vi "libssh2_knownhost_get - invalid known hosts collection - returns invalid host.vi"() -> ()   [LabVIEW 2013, in "libssh2_tests.lvlib"]
uses:
  libssh2_tests.lvlib
  libssh2/Known Host Collection Refnum.ctl
  libssh2/libssh2_init_default.vi
  <vilib>/addons/_JKI Toolkits/Caraya/classes/Assert/Assert True.vi
  <vilib>/addons/_JKI Toolkits/Caraya/classes/Test/Test.lvclass
  libssh2/libssh2.lvlib
  <vilib>/addons/_JKI Toolkits/Caraya/classes/Assert/Assert.lvclass
panel:
  out "error out":errorcluster
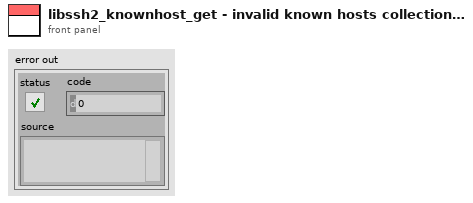
[diagram p1: front panel]
types:
  T1 = typedef "libssh2.lvlib/Session Refnum.ctl" = refnum<k1>
  T2 = typedef "libssh2.lvlib/Known Host Collection Refnum.ctl" = refnum<k1>
  T3 = typedef "libssh2.lvlib/Known Host Refnum.ctl" = refnum<k1>
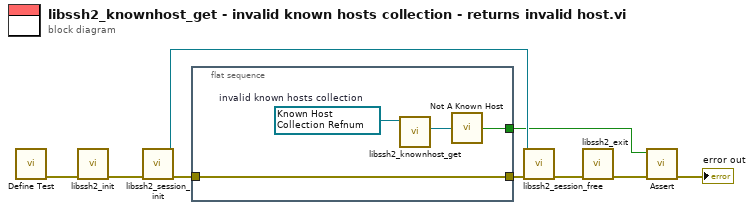
[diagram p0: block diagram]
diagram:
  n1 = call <vilib>:"Define Test.vi"() -> ("error out"=w8:errorcluster)  [unwired: 10 in, 1 out]
  n2 = call-poly "libssh2_init.vi"("error in (no error)"=w8) -> ("error out"=w7:errorcluster)  [unwired: 10 in]
  n3 = call "libssh2_session_init.vi"("error in (no error)"=w7) -> ("error out"=w1:errorcluster, "session"=w4:T1)  [unwired: 9 in]
  n4 = flat-sequence {
    tunnel: [w13] -> w3
    tunnel: [w12] -> w2
    tunnel: w1 -> [w12]
    frame #0 {
      w11 = T2 refnum items=["Known Hosts"]  # invalid known hosts collection
      n5 = call "libssh2_knownhost_get.vi"("known hosts collection"=w11) -> ("next"=w10:T3)  [unwired: 8 in, 2 out]
      n6 = call "Not A Known Host.vi"("known host"=w10) -> ("Not a Known Host?"=w13:bool)
    }
  }
  n7 = call "libssh2_session_free.vi"("error in (no error)"=w2, "session"=w4) -> ("error out"=w6:errorcluster)  [unwired: 9 in]
  n8 = call "libssh2_exit.vi"("error in (no error)"=w6) -> ("error out"=w5:errorcluster)  [unwired: 10 in]
  n9 = call-poly <vilib>:"Assert.vi"("error in (no error)"=w5, "True?"=w3) -> ("error out"=→"error out":errorcluster)  [unwired: 8 in, 1 out]
